vi "GPIB_OPC-check.vi"(1 "error out 2":errorcluster, 3 "GPIB Address":string) -> (0 "error out":errorcluster)   [LabVIEW 2013]
panel:
  in  "stop":bool
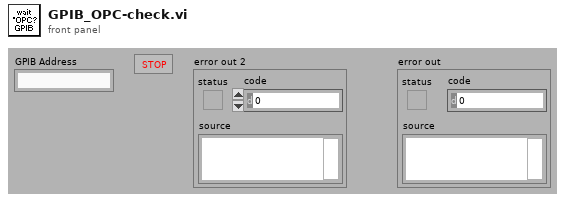
[diagram p1: front panel]
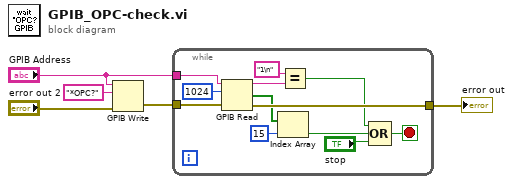
[diagram p0: block diagram]
diagram:
  n1 = GPIB Write(0:"GPIB Address", 1:"*OPC?" ("data"), 3:"error out 2") -> (6:w1:errorcluster)  [unwired: 3 out]
  n2 = while {
    tunnel: "GPIB Address" -> [w16]
    tunnel: w1 -> [w14]
    tunnel: [w15] -> w5
    stop <- w13 stop-if-true
    n3 = GPIB Read(0:w16, 1:1024 ("byte count"), 3:w14) -> (5:w11:string, 6:w9:bool[], 7:w15:errorcluster)  [unwired: 2 out]
    n4 = Index Array(array=w9, index=15) -> (element=w7:bool)
    n5 = Equal?(x="1\n", y=w11) -> (x = y?=w6:bool)
    n6 = Compound Arithmetic op=OR(w6, w7, "stop") -> (w13:bool)
  }
  "error out" <- w5
